vi "TrajTrimAnkleTrajAtEnd.vi"(2 "AnkleTraj":dbl[][](array[numeric]), 3 "Direction (x)":T1) -> (0 "AnkleTraj Leftover":dbl[][](array[numeric]), 1 "AnkleTraj Trimed":dbl[][](array[numeric]))   [LabVIEW 2016, in "ForceField.lvclass"]
doc: "Trim ankle trajectory at the forward most point (default is X direction)"
uses:
  ForceField.lvclass
  SerialChain/TypeDef/xyzO.ctl
  SerialChain/SerialChain.lvclass
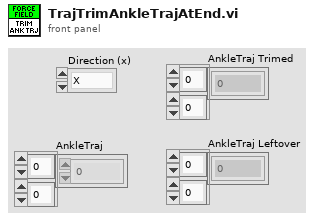
[diagram p1: front panel]
types:
  T1 = typedef "SerialChain.lvclass/xyzO.ctl" = enum16{"X", "Y", "Z", "O"}
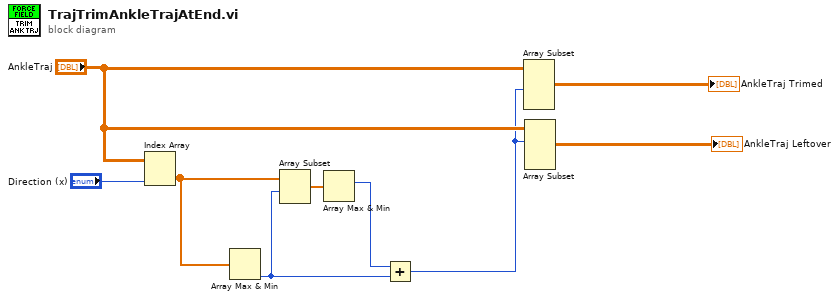
[diagram p0: block diagram]
diagram:
  n1 = Index Array(array="AnkleTraj", index (col)="Direction (x)") -> (element=w8:dbl[])  [unwired: 1 in]
  n2 = Array Max & Min(array=w8) -> (min index (indices)=w1:i32)  [unwired: 3 out]
  n3 = Array Subset(array=w8, index=w1) -> (w9:dbl[])  [unwired: 1 in]
  n4 = Array Max & Min(array=w9) -> (max index (indices)=w2:i32)  [unwired: 3 out]
  n5 = Add(x=w2, y=w1) -> (x+y=w4:i32)
  n6 = Array Subset(array="AnkleTraj", length (row)=w4) -> (→"AnkleTraj Trimed":dbl[][])  [unwired: 3 in]
  n7 = Array Subset(array="AnkleTraj", index (row)=w4) -> (→"AnkleTraj Leftover":dbl[][])  [unwired: 3 in]
